vi "Drag Start.vi"(8 "error in (no error)":errorcluster, 11 "BetterBoxHandle in":refnum<class "BetterBoxHandle.lvclass">) -> (0 "error out":errorcluster, 2 "BetterDropOp":refnum<class "BetterDropOp.lvclass">, 3 "BetterBoxHandle out":refnum<class "BetterBoxHandle.lvclass">)   [LabVIEW 2020, in "BetterDragAndDrop.lvlib" / "BetterBoxHandle.lvclass"]
uses:
  BetterBoxHandle.lvclass
  BetterDropOp/BetterDropOp.lvclass
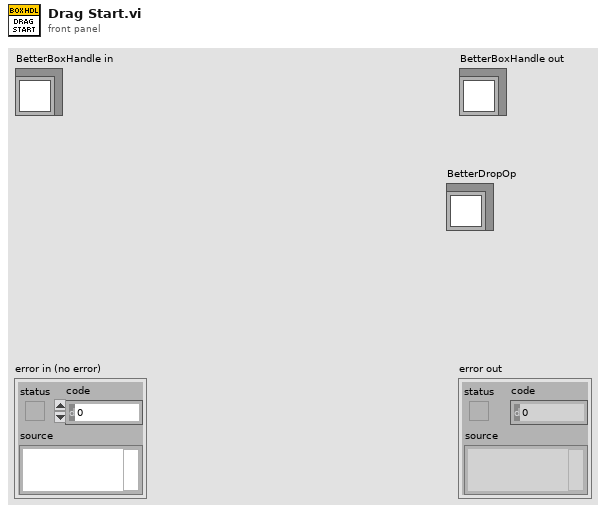
[diagram p1: front panel]
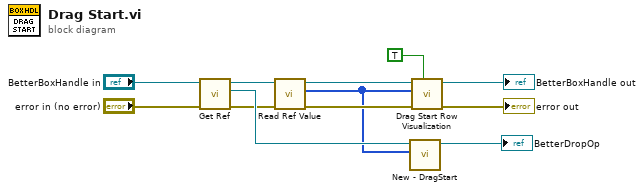
[diagram p0: block diagram]
diagram:
  n1 = call-dynamic "Get Ref.vi"("error in (no error)"="error in (no error)", "BetterHandle in"="BetterBoxHandle in") -> ("error out"=w9:errorcluster, "Tree/LB/MCL ref"=w10:refnum<vi>, "BetterHandle out"=w11:refnum<class "BetterBoxHandle.lvclass">)  [unwired: 7 in]
  n2 = call-dynamic "Read Ref Value.vi"("error in (no error)"=w9, "BetterBoxHandle in"=w11) -> ("error out"=w3:errorcluster, "Value"=w2:i32[], "BetterBoxHandle out"=w6:refnum<class "BetterBoxHandle.lvclass">)  [unwired: 7 in]
  n3 = call "New - DragStart.vi"("DragStart Indices"=w2, "Ref"=w10) -> ("BetterDropOp out"=→"BetterDropOp":refnum<class "BetterDropOp.lvclass">)  [unwired: 8 in, 1 out]
  n4 = call-dynamic "Drag Start Row Visualization.vi"("DragStart? (F)"=TRUE, "error in (no error)"=w3, "DragStart Indices"=w2, "BetterBoxHandle in"=w6) -> ("error out"=→"error out":errorcluster, "BetterBoxHandle out"=→"BetterBoxHandle out":refnum<class "BetterBoxHandle.lvclass">)  [unwired: 6 in]
